vi "PPs to RPM.vi"(6 "PPR":dbl=32.0 format="%#_13g", 8 "error in (no error)":errorcluster, 10 "Speed (Hz)":dbl) -> (0 "error out":errorcluster, 3 "RPM":dbl format="%0.2f")   [LabVIEW 2018]
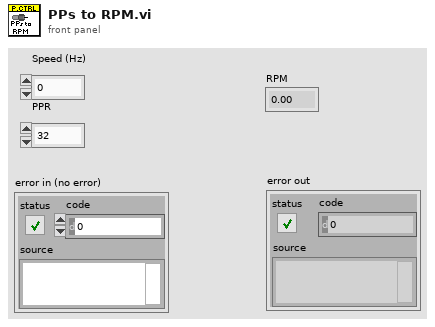
[diagram p1: front panel]
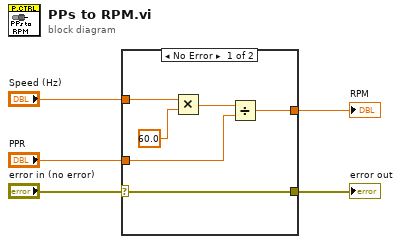
[diagram p0: block diagram]
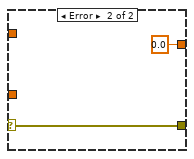
[diagram p2: hidden frame]
diagram:
  n1 = case shown="No Error" "error in (no error)" {
    selector: "error in (no error)" -> [w6 w13]
    tunnel: [w11 0.0] -> w5
    tunnel: "PPR" -> [w10 _]
    tunnel: "Speed (Hz)" -> [w7 _]
    tunnel: [w6 w13] -> w1
    frame No Error {
      n2 = Multiply(x=w7, y=60.0) -> (x*y=w9:dbl)
      n3 = Divide(x=w9, y=w10) -> (x/y=w11:dbl)
    }
    frame Error {
    }
  }
  "RPM" <- w5
  "error out" <- w1
